vi "Photon Counting.vi"() -> (13 "Frame acquisition finish?":bool)   [LabVIEW 2015]
uses:
  <vilib>/Platform/TimedLoop/XDataNode/timing_clust.ctl
  <vilib>/Platform/TimedLoop/XDataNode/nitl_modes.ctl
  <vilib>/Platform/TimedLoop/XDataNode/wakeup.ctl
  <vilib>/rvi/Emulation/niFpgaGetClockAttributes.vi
  <vilib>/rvi/Emulation/niFpgaSctlEmulationGetInTimedLoop.vi
  <vilib>/rvi/Emulation/niFpgaEmulationReportErrorSimple.vi
  <vilib>/rvi/Emulation/niFpgaCriticalErrorInLSC.vi
  Globals/Global Variable_Pixel Clock.vi
  <vilib>/rvi/Emulation/niFpgaProcessEmulError.vi
  Globals/Global_Sample per Frame.vi
  <vilib>/Platform/TimedLoop/XDataNode/XDataNode.xnode
  <vilib>/Platform/TimedLoop/XDataNode/XDNodeRunTimeDep.lvlib
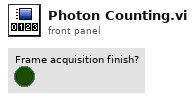
[diagram p1: front panel]
types:
  T1 = typedef "XDNodeRunTimeDep.lvlib/timing_clust.ctl" = cluster{"Expected End [f-1]":u64, "Actual End [f-1]":u64, "Finished Late? [f-1]":bool, "Expected End [i-1]":u64, "Actual End [i-1]":u64, "Finished Late? [i-1]":bool, "Expected Start [i]":u64, "Actual Start [i]":u64, "Expected Start [f]":u64, "Actual Start [f]":u64, "Source Name":string, "Structure Name":string, "Period":i64, "Deadline":i64, "Offset":i64, "Start":i64, "Priority":i32, "Timeout":i32, "Mode":T2, "Wakeup Reason":T3, "Error":errorcluster, "Source Type":string, "Secondary Source Type":string, "Global End Time":u64, "Global Start Time":u64, "Frame Duration":u64, "Iteration Duration":u64, "Assigned CPU":i32, "I/O Scan Engine Mode":u32}
  T2 = typedef "XDNodeRunTimeDep.lvlib/nitl_modes.ctl" = enum32{"No Change", "Process missed periods, maintain original phase", "Discard missed periods, maintain original phase", "Process missed periods, ignore original phase", "Discard missed periods, ignore original phase"}
  T3 = typedef "XDNodeRunTimeDep.lvlib/wakeup.ctl" = enum32{"Normal", "Aborted", "Asynchronous wakeup", "Timing source error", "Timed loop error", "Timeout"}
  T4 = cluster{"Numeric 1":u32, "Numeric 2":u32, "Numeric 3":u32, "Numeric 4":u32, "Numeric 5":u32, "Numeric 6":u32, "Numeric 7":u32, "Numeric 8":u32, "Numeric 9":u32, "Numeric 10":u32, "Numeric 11":u32, "Numeric 12":u32, "Numeric 13":u32, "Numeric 14":u32, "Numeric 15":u32, "Numeric 16":u32}
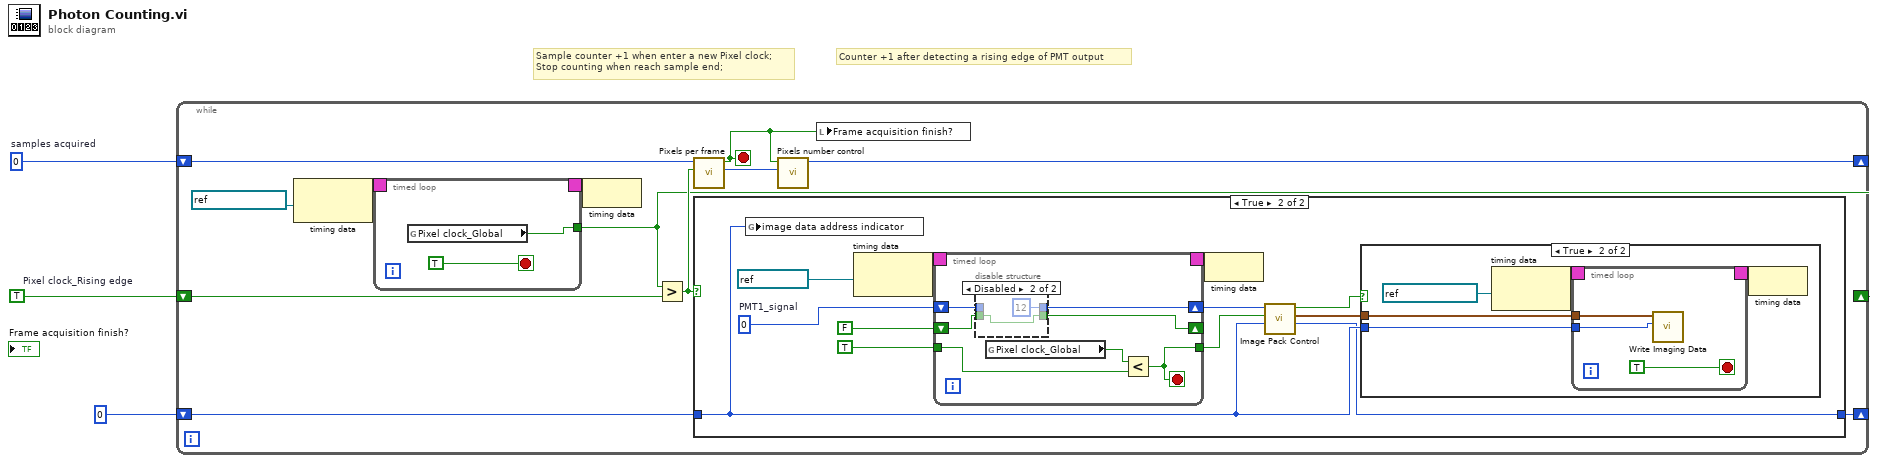
[diagram p0: block diagram]
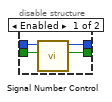
[diagram p4: hidden frame]
diagram:
  w2 = u32 0  # samples acquired
  w3 = TRUE  # Pixel clock_Rising edge
  # "Sample counter +1 when enter a new Pixel clock;\nStop counting when reach sample end;"
  # "Counter +1 after detecting a rising edge of PMT output"
  n1 = while {
    shift-right: [w4] -> _
    shift-left: w3 -> [w15]
    shift-right: [w7] -> _
    shift-left: w2 -> [w14]
    shift-right: [w5] -> _
    shift-left: u32 0 -> [w6]
    stop <- w9 stop-if-true
    n2 = node-c288(refnum<k21> "DRAM Clock" ("Source Name")) -> (w13:T1)
    n3 = timed-loop {
      timing: w13 -> [_]
      timing-out: [_] -> w12
      tunnel: [w16] -> w4
      stop <- TRUE stop-if-true
      n4 = global read "Global Variable_Pixel Clock.vi" "Pixel clock_Global"() -> (w16:bool)
    }
    n5 = node-c288(w12) -> ()
    n6 = Greater?(x=w4, y=w15) -> (0:w11:bool)
    n7 = call "Pixels per frame.vi"("Rising edge"=w11, ">> # of pixels collected in a frame >>"=w14) -> ("samples acquired"=w8:u32, "Boolean out"=w9:bool)  [unwired: 8 in]
    n8 = case shown="True" w11 {
      tunnel: w6 -> [w24 w29]
      tunnel: [w24 w28] -> w5
      frame False {
      }
      frame True {
        w34 = u16 0  # PMT1_signal
        n9 = global write "Global_Sample per Frame.vi" "image data address indicator"(w29) -> ()
        n10 = node-c288(refnum<k21> "280MHz" ("Photon counting rate")) -> (w36:T1)
        n11 = timed-loop {
          timing: w36 -> [_]
          timing-out: [_] -> w35
          shift-right: [w56] -> w30
          shift-left: w34 -> [w57]
          tunnel: TRUE -> [w52]
          tunnel: [w51] -> w31
          shift-right: [w54] -> _
          shift-left: FALSE ("y") -> [w55]
          stop <- w51 stop-if-true
          n12 = disable-structure shown="Disabled" {
            disable-tunnel: w57 -> [w61 _]
            disable-tunnel: [w60 u16 12 ("PMT1_signal out")] -> w56
            disable-tunnel: w55 -> [w59 w62]
            disable-tunnel: [w58 w62] -> w54
            frame Enabled {
              n13 = call "Signal Number Control.vi"("Previous PMT1"=w59, "PMT1_signal in"=w61) -> ("IO Module\\PMT1"=w58:bool, "PMT1_signal out"=w60:u16)  [unwired: 8 in]
            }
            frame Disabled {
            }
          }
          n14 = global read "Global Variable_Pixel Clock.vi" "Pixel clock_Global"() -> (w53:bool)
          n15 = Less?(x=w53, y=w52) -> (x < y?=w51:bool)
        }
        n16 = node-c288(w35) -> ()
        n17 = call "Image Pack Control.vi"("Numeric in"=w29, "input valid"=w31, "PMT1_signal"=w30) -> ("Numeric out"=w28:u32, "packer out"=w25:T4, "output valid?"=w27:bool)  [unwired: 6 in]
        n18 = case shown="True" w27 {
          tunnel: w29 -> [_ w38]
          tunnel: w25 -> [_ w37]
          frame False {
          }
          frame True {
            n19 = node-c288(refnum<k21> "DRAM Clock" ("Source Name")) -> (w41:T1)
            n20 = timed-loop {
              timing: w41 -> [_]
              timing-out: [_] -> w40
              tunnel: w38 -> [w44]
              tunnel: w37 -> [w43]
              stop <- TRUE stop-if-true
              n21 = call "Write Imaging Data.vi"("Address"=w44, "packer out"=w43) -> ()  [unwired: 10 in]
            }
            n22 = node-c288(w40) -> ()
          }
        }
      }
    }
    n23 = call "Pixels number control.vi"("samples acquired in"=w8, "Done?"=w9) -> ("samples acquired out"=w7:u32)  [unwired: 9 in]
    n24 = local write "Frame acquisition finish?"(w9) -> ()
  }
